vi "Configure Camera Parameters.vi"(8 "error in (no error)":errorcluster, 10 "parameters":T1 {"prechanrge bus" items=["no", "yes"]; "Y read mode" items=["forward", "backward"]; "X read mode" items=["forward", "backward"]; "CCD advanced mode" items=["none", "nondestructive", "double slope"]; "CCD mode" items=["parallel", "serial", "low dark current", "large full well"]; "OUT2 mode" items=["exposure (negative)", "exposure (positive)", "delay before esposure (negative)", "delay after esposure (negative)", "external input inverted", "external input", "user register bit 1", "software start scan", "reserved"]; "OUT1 mode" items=["exposure (negative)", "exposure (positive)", "delay before esposure (negative)", "delay after esposure (negative)", "external input inverted", "external input", "user register bit 0", "software start scan", "reserved"]; "synchronization mode" items=["software"=0, "hardware"=1, "external rising edge type 1"=2, "external rising edge type 2"=3, "external falling edge type 1"=10, "external falling edge type 2"=11]; "bits per pixel" items=["8", "10", "12", "14", "16"]}, 11 "SOL Camera in":refnum<class "PL SOL Instruments Camera.lvclass">) -> (0 "error out":errorcluster, 3 "SOL Camera out":refnum<class "PL SOL Instruments Camera.lvclass">)   [LabVIEW 2015, in "PL SOL Instruments Camera.lvclass"]
doc: "Configures camera parameters."
uses:
  PL SOL Instruments Camera.lvclass
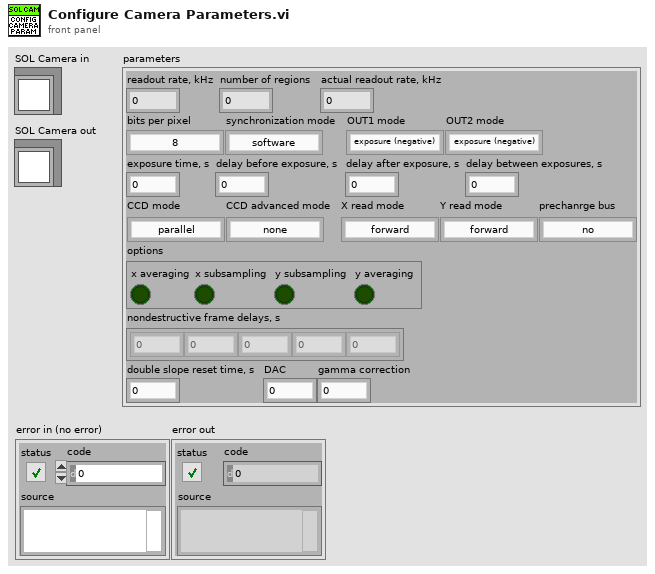
[diagram p1: front panel]
types:
  T1 = cluster{"number of regions":i32, "readout rate, kHz":i32, "actual readout rate, kHz":i32, "bits per pixel":u16, "synchronization mode":u16, "OUT1 mode":u16, "OUT2 mode":u16, "exposure time, s":dbl, "delay before exposure, s":dbl, "delay after exposure, s":dbl, "delay between exposures, s":dbl, "CCD mode":u16, "CCD advanced mode":u16, "X read mode":u16, "Y read mode":u16, "prechanrge bus":u16, "options":cluster{"x averaging":bool, "x subsampling":bool, "y subsampling":bool, "y averaging":bool}, "nondestructive frame delays, s":dbl[], "double slope reset time, s":dbl, "DAC":u16, "gamma correction":u16}
  T2 = cluster{"x averaging":bool, "x subsampling":bool, "y subsampling":bool, "y averaging":bool}
  T3 = cluster{"number of regions":i32, "readout rate, kHz":i32, "actual readout rate, kHz":i32, "bits per pixel":u16, "synchronization mode":u16, "OUT1 mode":u16, "OUT2 mode":u16}
  T4 = cluster{"CCD mode":u16, "CCD advanced mode":u16, "X read mode":u16, "Y read mode":u16, "prechanrge bus":u16, u16}
  T5 = cluster{"unit":u16, "value":u16, "DAC":u16, "gamma correction":u16}
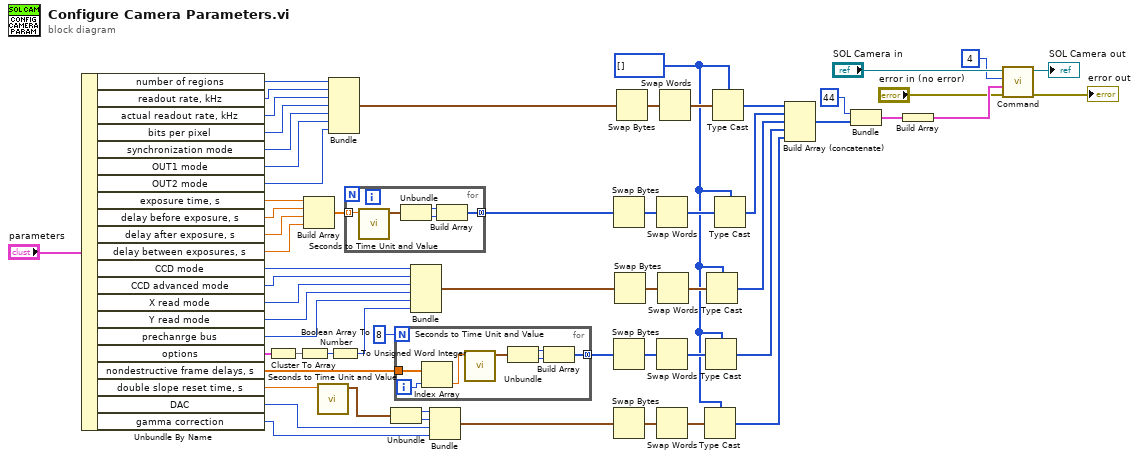
[diagram p0: block diagram]
diagram:
  w14 = u8[] [] ("response")
  n1 = Unbundle By Name("parameters") -> ("number of regions"=w60:i32, "readout rate, kHz"=w59:i32, "actual readout rate, kHz"=w58:i32, "bits per pixel"=w57:u16, "synchronization mode"=w56:u16, "OUT1 mode"=w55:u16, "OUT2 mode"=w54:u16, "exposure time, s"=w53:dbl, "delay before exposure, s"=w52:dbl, "delay after exposure, s"=w51:dbl, "delay between exposures, s"=w50:dbl, "CCD mode"=w38:u16, "CCD advanced mode"=w37:u16, "X read mode"=w36:u16, "Y read mode"=w35:u16, "prechanrge bus"=w34:u16, "options"=w41:T2, "nondestructive frame delays, s"=w27:dbl[], "double slope reset time, s"=w2:dbl, "DAC"=w19:u16, "gamma correction"=w18:u16)
  n2 = Cluster To Array(cluster=w41) -> (array=w40:bool[])
  n3 = Boolean Array To Number(Boolean array=w40) -> (number=w39:u32)
  n4 = Build Array(w53, w52, w51, w50) -> (w49:dbl[])
  n5 = call "Seconds to Time Unit and Value.vi"("time, s"=w2) -> ("time unit and value"=w1:cluster{"unit":u16, "value":u16})  [unwired: 10 in]
  n6 = Bundle("number of regions"=w60, "readout rate, kHz"=w59, "actual readout rate, kHz"=w58, "bits per pixel"=w57, "synchronization mode"=w56, "OUT1 mode"=w55, "OUT2 mode"=w54) -> (w47:T3)  [unwired: 1 in]
  n7 = To Unsigned Word Integer(number=w39) -> (unsigned 16bit integer=w33:u16)
  n8 = for {
    tunnel: w49 -> [w62] mode=indexing
    tunnel: [w63] -> w45 mode=concatenating
    n9 = call "Seconds to Time Unit and Value.vi"("time, s"=w62) -> ("time unit and value"=w61:cluster{"unit":u16, "value":u16})  [unwired: 10 in]
    n10 = Unbundle(w61) -> ("unit"=w64:u16, "value"=w65:u16)
    n11 = Build Array(w64, w65) -> (w63:u16[])
  }
  n12 = Unbundle(w1) -> ("unit"=w21:u16, "value"=w20:u16)
  n13 = for {
    N: 8 -> [_]
    tunnel: w27 -> [w72]
    tunnel: [w68] -> w24 mode=concatenating
    i -> [w71]
    n14 = Index Array(array=w72, index=w71) -> (element=w66:dbl)
    n15 = call "Seconds to Time Unit and Value.vi"("time, s"=w66) -> ("time unit and value"=w67:cluster{"unit":u16, "value":u16})  [unwired: 10 in]
    n16 = Unbundle(w67) -> ("unit"=w70:u16, "value"=w69:u16)
    n17 = Build Array(w70, w69) -> (w68:u16[])
  }
  n18 = Bundle("CCD mode"=w38, "CCD advanced mode"=w37, "X read mode"=w36, "Y read mode"=w35, "prechanrge bus"=w34, w33) -> (w31:T4)  [unwired: 1 in]
  n19 = Bundle("unit"=w21, "value"=w20, "DAC"=w19, "gamma correction"=w18) -> (w16:T5)  [unwired: 1 in]
  n20 = Swap Bytes(anything=w45) -> (byte swapped=w46:u16[])
  n21 = Swap Bytes(anything=w24) -> (byte swapped=w25:u16[])
  n22 = Swap Bytes(anything=w16) -> (byte swapped=w17:T5)
  n23 = Swap Bytes(anything=w31) -> (byte swapped=w32:T4)
  n24 = Swap Bytes(anything=w47) -> (byte swapped=w48:T3)
  n25 = Swap Words(1:w46) -> (0:w42:u16[])
  n26 = Swap Words(1:w25) -> (0:w23:u16[])
  n27 = Swap Words(1:w17) -> (0:w15:T5)
  n28 = Swap Words(1:w32) -> (0:w30:T4)
  n29 = Swap Words(1:w48) -> (0:w44:T3)
  n30 = Type Cast(type=w14, x=w15) -> (*(type *) &x=w13:u8[])
  n31 = Type Cast(type=w14, x=w23) -> (*(type *) &x=w22:u8[])
  n32 = Type Cast(type=w14, x=w30) -> (*(type *) &x=w28:u8[])
  n33 = Type Cast(type=w14, x=w44) -> (*(type *) &x=w43:u8[])
  n34 = Type Cast(type=w14, x=w42) -> (*(type *) &x=w29:u8[])
  n35 = Build Array (concatenate)(w43, w29, w28, w22, w13) -> (w10:u8[])
  n36 = Bundle("offset"=44, w10) -> (w11:cluster{"offset":i32, u8[]})  [unwired: 1 in]
  n37 = Build Array(w11) -> (w5:cluster{"offset":i32, u8[]}[])
  n38 = call "Command.vi"("error in (no error)"="error in (no error)", "data"=w5, "command"=u8 4, "SOL Camera in"="SOL Camera in") -> ("error out"=→"error out":errorcluster, "SOL Camera out"=→"SOL Camera out":refnum<class "PL SOL Instruments Camera.lvclass">)  [unwired: 5 in, 1 out]
